vi "update diagnostic channel.vi"(5 "report?":bool, 7 "Channel Name?":string, 8 "error in":errorcluster, 9 "Selected Slave":i8, 10 "engine configuration in":refnum<class "engine configuration.lvclass">, 11 "Profibus Module editor node in":refnum<class "Profibus Module editor node.lvclass">) -> (0 "error out":errorcluster, 1 "new chan name":string, 2 "engine configuration out":refnum<class "engine configuration.lvclass">, 3 "Profibus Module editor node out":refnum<class "Profibus Module editor node.lvclass">)   [LabVIEW 2013, in "Profibus Module editor node.lvclass"]
uses:
  Profibus Module editor node.lvclass
  <vilib>/NI/Module Execution Interface/Engine Configuration/engine configuration.lvclass
  Profibus Module editor node.lvclass/Profibus Module editor node.ctl
  <vilib>/NI/TBM Modules/Profibus/configuration/Profibus Module configuration.lvclass/Profibus Module configuration.ctl
  <vilib>/NI/Tag Bus Module Framework/root configuration/TBM configuration.lvclass/TBM configuration.ctl
  <vilib>/NI/Tag Bus Module Framework/channel/TBM channel.lvclass
  <vilib>/NI/Tag Bus/tag/Data Type.ctl
  <vilib>/NI/Tag Bus Module Framework/channel/channel classification.ctl
  <vilib>/NI/Tag Bus/tag/tag descriptor.lvclass/tag descriptor.ctl
  <vilib>/NI/Tag Bus Module Framework/root configuration/create GUID.vi
  <vilib>/NI/TBM Modules/Profibus/configuration/Profibus Module configuration.lvclass
  <vilib>/NI/Tag Bus Module Framework/root configuration/TBM configuration.lvclass
  <vilib>/NI/Tag Bus/tag/tag descriptor.lvclass
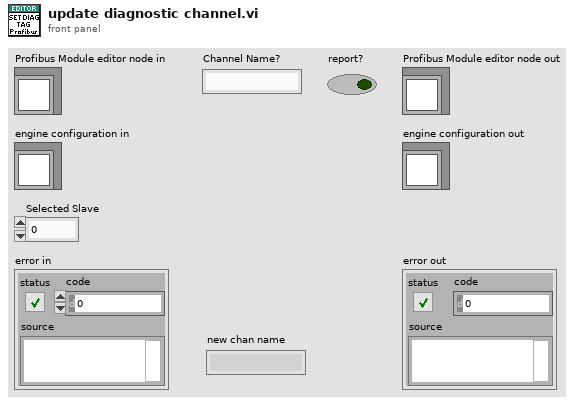
[diagram p1: front panel]
types:
  T1 = typedef "Profibus Module configuration.lvclass/slave diagnostic configuration.ctl" = cluster{"slave":i8, "report":bool, "channel":refnum<class "TBM channel.lvclass">, "error specs":T2[]}
  T2 = typedef "Profibus Module configuration.lvclass/error throw specification.ctl" = cluster{"byte":i32, "bit":i32, "inverted?":bool, "error":i32}
  T3 = typedef "TBM channel.lvclass/channel classification.ctl" = enum16{"input data", "output data", "processing parameter", "processing result"}
  T4 = typedef "tag bus.lvlib/tag descriptor.lvclass/Data Type.ctl" = enum16{"Double", "Single", "I64", "I32", "I16", "I8", "U64", "U32", "U16", "U8", "Boolean", "String", "Array of Double", "Array of Single", "Array of I64", "Array of I32", "Array of I16", "Array of I8", "Array of U64", "Array of U32", "Array of U16", "Array of U8", "Array of Boolean", "Array of String"}
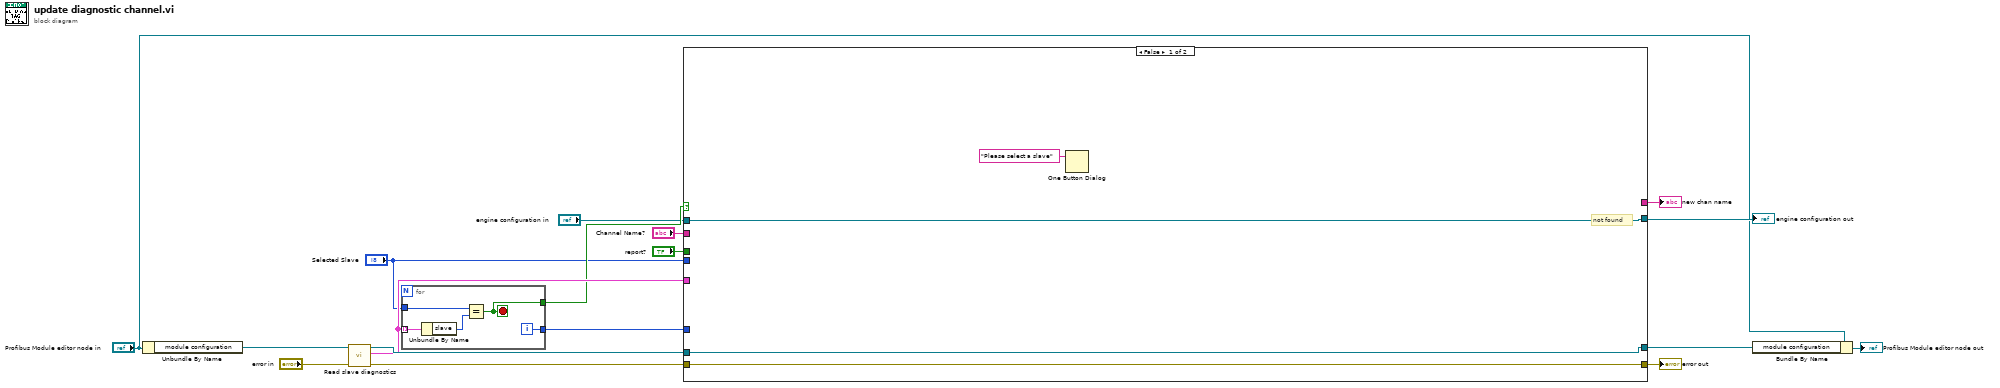
[diagram p0: block diagram]
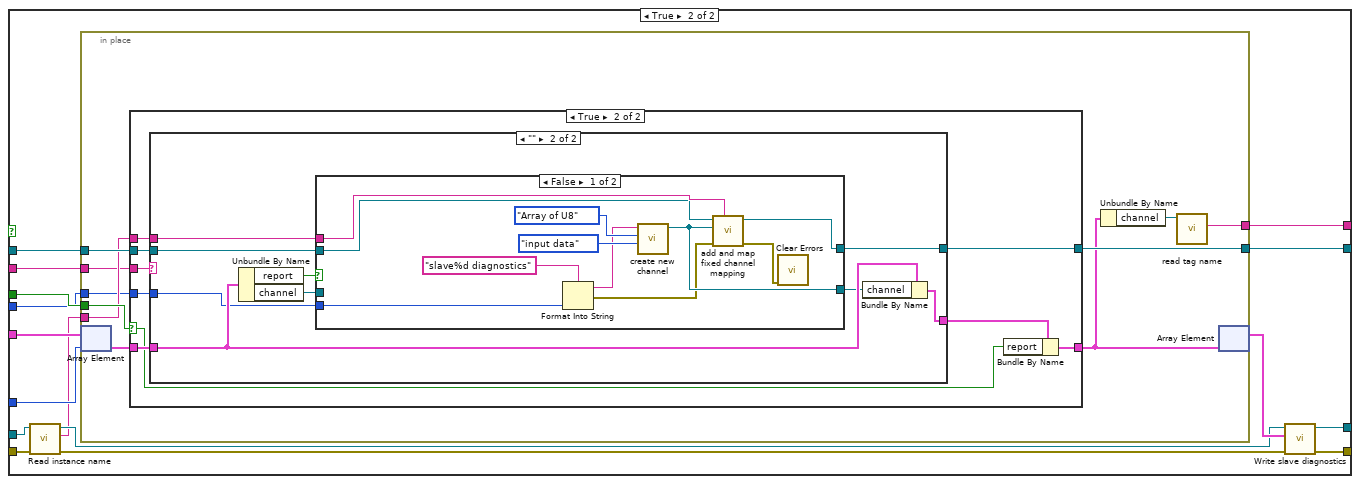
[diagram p2: hidden frame]
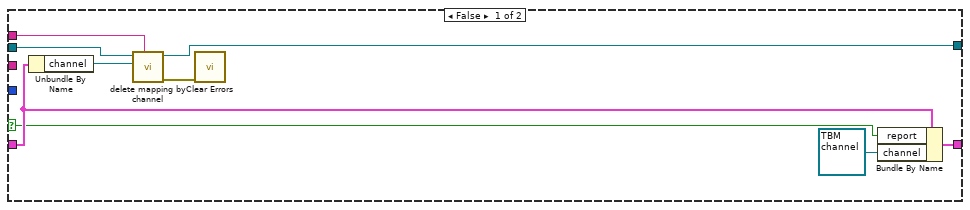
[diagram p3: hidden frame]
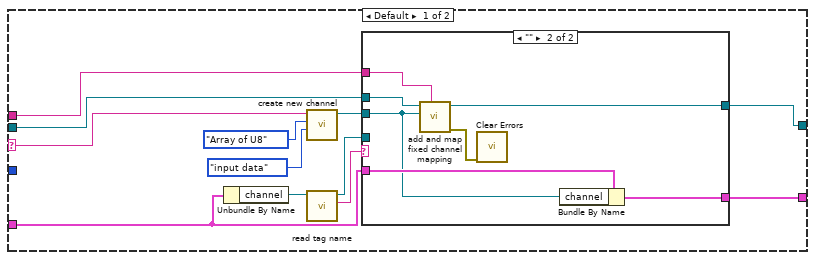
[diagram p4: hidden frame]
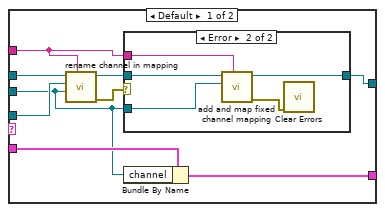
[diagram p5: hidden frame]
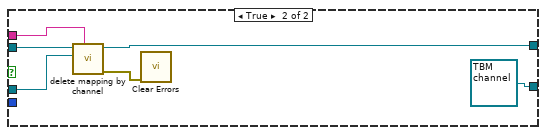
[diagram p7: hidden frame]
diagram:
  n1 = Unbundle By Name("Profibus Module editor node in") -> ("module configuration"=w6:refnum<class "Profibus Module configuration.lvclass">)
  n2 = call <vilib>:"Read slave diagnostics.vi"("error in"="error in", "Profibus Module configuration in"=w6) -> ("error out"=w8:errorcluster, "slave diagnostics"=w12:T1[], "Profibus Module configuration out"=w15:refnum<class "Profibus Module configuration.lvclass">)  [unwired: 7 in]
  n3 = for {
    tunnel: w12 -> [w22] mode=indexing
    tunnel: "Selected Slave" -> [w20]
    tunnel: [w19] -> w9
    tunnel: [w18] -> w10
    i -> [w18]
    stop <- w19 stop-if-true
    n4 = Unbundle By Name(w22) -> ("slave"=w21:i8)
    n5 = Equal?(x=w20, y=w21) -> (x = y?=w19:bool)
  }
  n6 = case shown="False" w9 {
    tunnel: w8 -> [w26 w41]
    tunnel: w10 -> [_ w37]
    tunnel: [w26 w40] -> w11
    tunnel: w12 -> [_ w38]
    tunnel: w15 -> [w25 w32]
    tunnel: [w25 w39] -> w16
    tunnel: "engine configuration in" -> [w24 w35]
    tunnel: [w24 w34] -> w17
    tunnel: "report?" -> [_ w42]
    tunnel: "Channel Name?" -> [_ w29]
    tunnel: [_ w28] -> w2
    tunnel: "Selected Slave" -> [_ w27]
    frame False {
      # "not found"
      n7 = One Button Dialog(message="Please select a slave") -> ()  [unwired: 1 in, 1 out]
    }
    frame True {
      n8 = call <vilib>:"Read instance name.vi"("error in"=w41, "configuration in"=w32) -> ("error out"=w33:errorcluster, "instance id"=w30:string, "configuration out"=w31:refnum<class "Profibus Module configuration.lvclass">)  [unwired: 7 in]
      n9 = in-place {
        in-place-border: w42 -> [w52]
        in-place-border: w35 -> [w51]
        in-place-border: [w50] -> w34
        in-place-border: w30 -> [w48]
        in-place-border: w29 -> [w47]
        in-place-border: [w44] -> w28
        in-place-border: w27 -> [w43]
        n10 = in-place-array #1(w38, w37) -> (w49:T1)
        n11 = case shown="True" w52 {
          selector: w52 -> [w58 w63]
          tunnel: w51 -> [w55 w67]
          tunnel: [w56 w66] -> w50
          tunnel: w49 -> [w60 w69]
          tunnel: [w59 w64] -> w46
          tunnel: w48 -> [w54 w68]
          tunnel: w47 -> [_ w70]
          tunnel: w43 -> [_ w62]
          frame False {
            n12 = Unbundle By Name(w60) -> ("channel"=w61:refnum<class "TBM channel.lvclass">)
            n13 = call <vilib>:"delete mapping by channel.vi"("owner ID"=w54, "channel"=w61, "engine configuration in"=w55) -> ("error out"=w53:errorcluster, "engine configuration out"=w56:refnum<class "engine configuration.lvclass">)  [unwired: 7 in]
            n14 = call <vilib>:"Clear Errors.vi"("error in (no error)"=w53) -> ()  [unwired: 6 in, 1 out]
            n15 = Bundle By Name(cluster=w60, "report"=w58, "channel"=refnum<class "TBM channel.lvclass"> refnum) -> (w59:T1)
          }
          frame True {
            n16 = case shown="\"\"" w70 {
              selector: w70 -> [w77 _]
              tunnel: w69 -> [w73 w113]
              tunnel: w68 -> [w78 w112]
              tunnel: w67 -> [w80 w111]
              tunnel: [w79 w110] -> w66
              tunnel: [w72 w109] -> w65
              tunnel: w62 -> [_ w105]
              frame Default {
                n17 = Unbundle By Name(w73) -> ("channel"=w82:refnum<class "TBM channel.lvclass">)
                n18 = call <vilib>:"create new channel.vi"("channel classification"=channel_classification."input data", "data type"=Data_Type."Array of U8", "channel name"=w77) -> ("channel"=w76:refnum<class "TBM channel.lvclass">)  [unwired: 8 in]
                n19 = call <vilib>:"read tag name.vi"("system tag in"=w82) -> ("name"=w81:string, "system tag out"=w71:refnum<class "TBM channel.lvclass">)  [unwired: 8 in, 1 out]
                n20 = case shown="\"\"" w81 {
                  tunnel: w80 -> [w91 w104]
                  tunnel: [w86 w103] -> w79
                  tunnel: w78 -> [w84 w102]
                  tunnel: w76 -> [w83 w99]
                  tunnel: w73 -> [w89 w100]
                  tunnel: [w88 w98] -> w72
                  tunnel: w71 -> [w90 _]
                  frame Default {
                    n21 = call <vilib>:"rename channel in mapping.vi"("owner ID"=w84, "new channel"=w83, "old channel"=w90, "engine configuration in"=w91) -> ("error out"=w87:errorcluster, "engine configuration out"=w85:refnum<class "engine configuration.lvclass">)  [unwired: 6 in]
                    n22 = case shown="Error" w87 {
                      tunnel: [w92 w94] -> w86
                      tunnel: w85 -> [w92 w95]
                      tunnel: w84 -> [_ w96]
                      tunnel: w83 -> [_ w93]
                      frame No Error {
                      }
                      frame Error {
                        n23 = call <vilib>:"add and map fixed channel mapping.vi"("module instance"=w96, "fixed channel"=w93, "engine configuration in"=w95) -> ("error out"=w97:errorcluster, "engine configuration out"=w94:refnum<class "engine configuration.lvclass">)  [unwired: 7 in]
                        n24 = call <vilib>:"Clear Errors.vi"("error in (no error)"=w97) -> ()  [unwired: 6 in, 1 out]
                      }
                    }
                    n25 = Bundle By Name(cluster=w89, "channel"=w83) -> (w88:T1)
                  }
                  frame "" {
                    n26 = call <vilib>:"add and map fixed channel mapping.vi"("module instance"=w102, "fixed channel"=w99, "engine configuration in"=w104) -> ("error out"=w101:errorcluster, "engine configuration out"=w103:refnum<class "engine configuration.lvclass">)  [unwired: 7 in]
                    n27 = call <vilib>:"Clear Errors.vi"("error in (no error)"=w101) -> ()  [unwired: 6 in, 1 out]
                    n28 = Bundle By Name(cluster=w100, "channel"=w99) -> (w98:T1)
                  }
                }
              }
              frame "" {
                n29 = Unbundle By Name(w113) -> ("report"=w107:bool, "channel"=w108:refnum<class "TBM channel.lvclass">)
                n30 = case shown="False" w107 {
                  tunnel: w112 -> [w123 w129]
                  tunnel: w111 -> [w122 w128]
                  tunnel: [w124 w127] -> w110
                  tunnel: w108 -> [_ w126]
                  tunnel: [w119 refnum<class "TBM channel.lvclass"> refnum ("channel")] -> w106
                  tunnel: w105 -> [w117 _]
                  frame False {
                    n31 = Format Into String(format string="slave%d diagnostics", w117) -> (resulting string=w115:string, error out=w116:errorcluster)  [unwired: 2 in]
                    n32 = call <vilib>:"create new channel.vi"("channel classification"=channel_classification."input data", "data type"=Data_Type."Array of U8", "channel name"=w115) -> ("channel"=w119:refnum<class "TBM channel.lvclass">)  [unwired: 8 in]
                    n33 = call <vilib>:"add and map fixed channel mapping.vi"("module instance"=w123, "error in"=w116, "fixed channel"=w119, "engine configuration in"=w122) -> ("error out"=w118:errorcluster, "engine configuration out"=w124:refnum<class "engine configuration.lvclass">)  [unwired: 6 in]
                    n34 = call <vilib>:"Clear Errors.vi"("error in (no error)"=w118) -> ()  [unwired: 6 in, 1 out]
                  }
                  frame True {
                    n35 = call <vilib>:"delete mapping by channel.vi"("owner ID"=w129, "channel"=w126, "engine configuration in"=w128) -> ("error out"=w130:errorcluster, "engine configuration out"=w127:refnum<class "engine configuration.lvclass">)  [unwired: 7 in]
                    n36 = call <vilib>:"Clear Errors.vi"("error in (no error)"=w130) -> ()  [unwired: 6 in, 1 out]
                  }
                }
                n37 = Bundle By Name(cluster=w113, "channel"=w106) -> (w109:T1)
              }
            }
            n38 = Bundle By Name(cluster=w65, "report"=w63) -> (w64:T1)
          }
        }
        n39 = Unbundle By Name(w46) -> ("channel"=w45:refnum<class "TBM channel.lvclass">)
        n40 = call <vilib>:"read tag name.vi"("system tag in"=w45) -> ("name"=w44:string)  [unwired: 8 in, 2 out]
        n41 = in-place-array #1(w46) -> (w36:T1[])  [unwired: 1 out]
      }
      n42 = call <vilib>:"Write slave diagnostics.vi"("error in"=w33, "slave diagnostics"=w36, "Profibus Module configuration in"=w31) -> ("error out"=w40:errorcluster, "Profibus Module configuration out"=w39:refnum<class "Profibus Module configuration.lvclass">)  [unwired: 7 in]
    }
  }
  "error out" <- w11
  "engine configuration out" <- w17
  "new chan name" <- w2
  n43 = Bundle By Name(cluster="Profibus Module editor node in", "module configuration"=w16) -> (→"Profibus Module editor node out":refnum<class "Profibus Module editor node.lvclass">)
